vi "Actor Core.vi"(8 "error in":errorcluster, 11 "ViewableChart In":refnum<class "ViewableChart.lvclass">) -> (0 "error out":errorcluster, 3 "Actor out":refnum<class "Actor.lvclass">)   [LabVIEW 2017, in "ViewableChart.lvclass"]
doc: "(<B>Filename</B>: Actor Framework.lvlib:Actor.lvclass:Actor Core.vi)\n\nReceives messages to the actor, reacts to them, and initiates any error handling that may shut the actor down.\n\nDescendant classes may override this VI to append parallel tasks for the actor to complete while it handles messages. Overrides use the Call Parent Method node.\n\n<License>\nCopyright © 2017 Composed Systems, LLC | All rights reserved\nwww.composed.io\n\nAuthor: Ethan Stern <ethan.stern@composed.io>\n\nThis software is provided \"AS IS\" WITHOUT WARRANTIES, either express or implied, AND IS FOR EDUCATIONAL PURPOSES ONLY.\n</License>MVA Framework 1.7.0.33\nEthan Stern - Composed Systems\nCopyright (c) 2018, Composed Systems"
uses:
  <vilib>/gpm_packages/@cs/example/Dynamic Viewables/ViewableChart/ViewableChart.lvclass
  C:/Program Files/National Instruments/LabVIEW 2017/vi.lib/gpm_packages/@cs/mva-viewable/Source/IViewable/IViewable/IViewable.lvclass
  <vilib>/ActorFramework/Actor/Actor.lvclass
  <vilib>/gpm_packages/@cs/example/Dynamic Viewables/ViewableChart/ViewableChart.lvclass/ViewableChart.ctl
  <vilib>/gpm_packages/@cs/mva-viewable/Source/IViewable/IViewable/IViewable.lvclass
panel:
  out "Waveform Chart - Dark":dbl(graph) caption="Chart Caption"
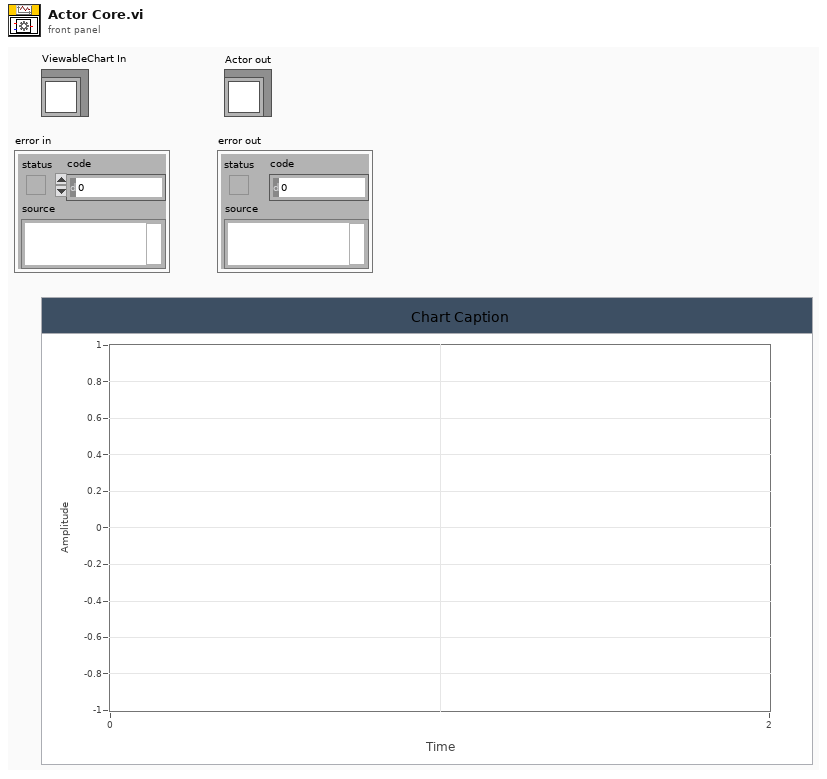
[diagram p1: front panel]
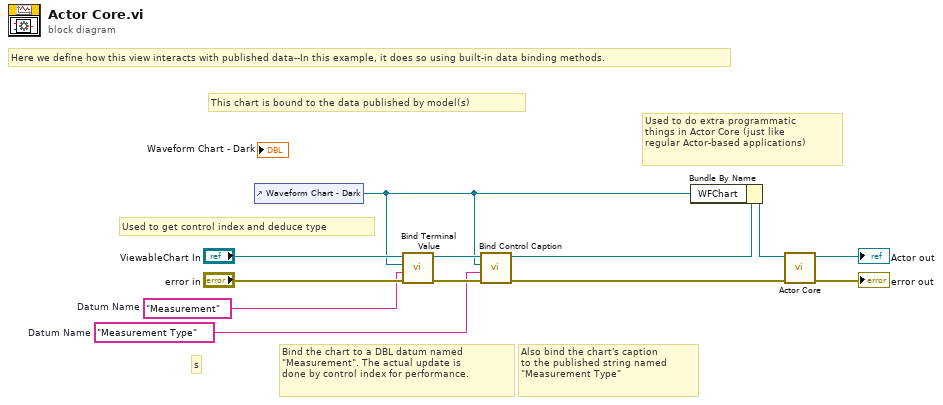
[diagram p0: block diagram]
diagram:
  w6 = "Measurement Type"  # Datum Name
  w1 = "Measurement"  # Datum Name
  # "s"
  # "Used to do extra programmatic\nthings in Actor Core (just like\nregular Actor-based applications)"
  # "Bind the chart to a DBL datum named\n\"Measurement\". The actual update is\ndone by control index for performance."
  # "Here we define how this view interacts with published data--In this example, it does so using built-in data binding methods."
  # "Also bind the chart's caption\nto the published string named\n\"Measurement Type\""
  # "Used to get control index and deduce type"
  # "This chart is bound to the data published by model(s)"
  n1 = control-ref of="Waveform Chart - Dark"() -> (w2:refnum<vi>)
  n2 = call <vilib>:"Bind Terminal Value.vi"("error in (no error)"="error in", "Datum Name (\"\"=Use Control Label)"=w1, "Ctl Refnum"=w2, "IViewable in"="ViewableChart In") -> ("error out"=w8:errorcluster, "IViewable out"=w7:refnum<class "ViewableChart.lvclass">)  [unwired: 6 in]
  n3 = call <vilib>:"Bind Control Caption.vi"("error in (no error)"=w8, "Datum Name (\"\"=Use Control Label)"=w6, "Control Refnum"=w2, "IViewable in"=w7) -> ("error out"=w3:errorcluster, "IViewable out"=w4:refnum<class "ViewableChart.lvclass">)  [unwired: 6 in]
  n4 = Bundle By Name(cluster=w4, "WFChart"=w2) -> (w5:refnum<class "ViewableChart.lvclass">)
  n5 = call-parent "Actor Core.vi"("error in"=w3, "IViewable In"=w5) -> ("error out"=→"error out":errorcluster, "Actor out"=→"Actor out":refnum<class "Actor.lvclass">)  [unwired: 8 in]
